vi "Read Profiles.vi"(8 "error in (no error)":errorcluster, 9 "Data Size (0: Auto Size)":u32, 10 "Read Req":T3 {"Profile Pos" items=["CURRENT", "OLDEST", "SPECIFY"]}, 11 "Device ID (0)":i32) -> (0 "error out":errorcluster, 1 "Profile Rsp":T2, 2 "Profile Data":u32[](array[numeric]), 3 "Device ID out":i32, 5 "Profile Info":T1)   [LabVIEW 2015, in "KEYENCE LJ-X8000A.lvlib"]
doc: "This function gets profile data.\nProfile data is stored in units of 0.01 ƒÊm.\nFor details on the data stored in the profile data (storage order and size), \nrefer to reference manual."
uses:
  KEYENCE LJ-X8000A.lvlib
  Clusters/Read Profile Req.ctl
  Constants/Profile Pos.ctl
  Clusters/Read Profile Rsp.ctl
  Clusters/Profile Info.ctl
panel:
  # "(c) 2019 KEYENCE CORPORATION.  ALL RIGHTS RESERVED."
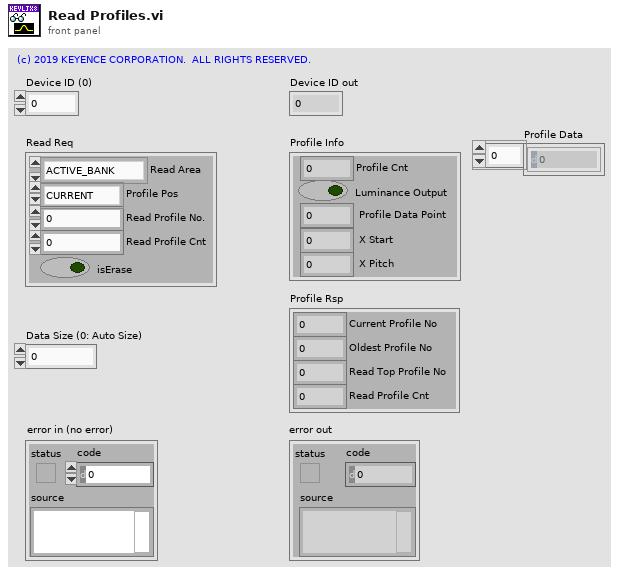
[diagram p1: front panel]
types:
  T1 = typedef "KEYENCE LJ-X8000A.lvlib/Profile Info.ctl" = cluster{"Profile Cnt":u8, "Luminance Output":bool, " Profile Data Point":u16, " X Start":i32, " X Pitch":i32}
  T2 = typedef "KEYENCE LJ-X8000A.lvlib/Read Profile Rsp.ctl" = cluster{"Current Profile No":u32, "Oldest Profile No":u32, "Read Top Profile No":u32, "Read Profile Cnt":u8}
  T3 = typedef "KEYENCE LJ-X8000A.lvlib/Read Profile Req.ctl" = cluster{"Read Area":enum8{"ACTIVE_BANK", "INACTIVE_BANK"}, "Profile Pos":T4, "Read Profile No.":u32, "Read Profile Cnt":u8, "isErase":bool}
  T4 = typedef "KEYENCE LJ-X8000A.lvlib/Profile Pos.ctl" = u8
  T5 = cluster{"Read Area":enum8{"ACTIVE_BANK", "INACTIVE_BANK"}, "Profile Pos":T4, "reserve":u8, "reserve":u8, "Read Profile No.":u32, "Read Profile Cnt":u8, "Erase":u8, "reserve":u8, "reserve":u8}
  T6 = cluster{"dwCurrentProfileNo":u32, "dwOldestProfileNo":u32, "dwGetTopProfileNo":u32, "byGetProfileCount":u8, "reserve":u8, "reserve":u8, "reserve":u8}
  T7 = cluster{"byProfileCount":u8, "reserve":u8, "byLuminanceOutput":u8, "reserve":u8, "wProfileDataCount":u16, "reserve":u8, "reserve":u8, "lXStart":i32, "lXPitch":i32}
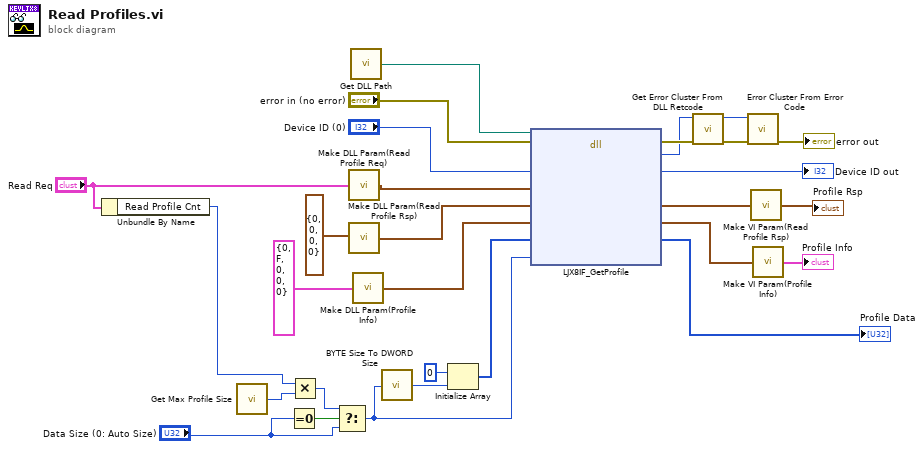
[diagram p0: block diagram]
diagram:
  n1 = Unbundle By Name("Read Req") -> ("Read Profile Cnt"=w17:u8)
  n2 = call "Get Max Profile Size.vi"() -> ("Profile Size"=w21:u32)  [unwired: 5 in]
  n3 = Equal To 0?(x="Data Size (0: Auto Size)") -> (x = 0?=w22:bool)
  n4 = Multiply(x=w17, y=w21) -> (x*y=w20:u32)
  n5 = Select(t=w20, s=w22, f="Data Size (0: Auto Size)") -> (s? t:f=w3:u32)
  n6 = call "Make DLL Param(Read Profile Req).vi"("Read Profile Req"="Read Req") -> ("DLL Read Profile Req"=w24:T5)
  n7 = call "Make DLL Param(Read Profile Rsp).vi"("Read Profile Rsp 2"=T2 {"Current Profile No"=0, "Oldest Profile No"=0, "Read Top Profile No"=0, "Read Profile Cnt"=0}) -> ("pRsp"=w12:T6)
  n8 = call "Get DLL Path.vi"() -> ("DLL Path"=w27:path)  [unwired: 3 in]
  n9 = call "Make DLL Param(Profile Info).vi"("Profile Info"=T1 {"Profile Cnt"=0, "Luminance Output"=FALSE, " Profile Data Point"=0, " X Start"=0, " X Pitch"=0}) -> ("DLL Parameter"=w10:T7)
  n10 = call "BYTE Size To DWORD Size.vi"("BYTE Size"=w3) -> ("DWORD Size"=w4:u32)
  n11 = Initialize Array(u32 0, w4) -> (w18:u32[])
  n12 = dll-call lib="C:/Program Files (x86)/National Instruments/LabVIEW 2018/instr.lib/KEYENCE LJ-X8000/LJX8_IF.*" fn="LJX8IF_GetProfile"(path in=w27, error in="error in (no error)", "lDeviceId"="Device ID (0)", "pReq"=w24, "pRsp"=w12, "pProfileInfo"=w10, "pdwProfileData"=w18, "dwDataSize"=w3) -> (error out=w16:errorcluster, "lRetCode"=w15:i32, "lDeviceId"=→"Device ID out":i32, "pRsp"=w8:T6, "pProfileInfo"=w6:T7, "pdwProfileData"=→"Profile Data":u32[])  [unwired: 3 in, 1 out]
  n13 = call "Get Error Cluster From DLL Retcode.vi"("error in (no error)"=w16, "DLL Return Code"=w15) -> ("error out"=w14:errorcluster, "VI Error Code"=w1:i32)  [unwired: 8 in]
  n14 = call <vilib>:"Error Cluster From Error Code.vi"("error in (no error)"=w14, "error code (0)"=w1) -> ("error out"=→"error out":errorcluster)  [unwired: 7 in]
  n15 = call "Make VI Param(Read Profile Rsp).vi"("pRsp"=w8) -> ("Read Profile Rsp"=→"Profile Rsp":T2)
  n16 = call "Make VI Param(Profile Info).vi"("pProfileInfo"=w6) -> ("Profile Info"=→"Profile Info":T1)
